vi "Basic Example.vi"() -> ()   [LabVIEW 2020]
uses:
  Laser Parameters.vi
panel:
  in  "REST port":string="35100"
  in  "Laser IP":string="10.0.40.83"
  in  "Ch2 Shutter":bool
  in  "Set Ch2 Wavl":bool
  in  "Ch2 Wavelength (nm)":dbl caption="Wavelength"
  in  "Ch1 Shutter":bool
  in  "Set Ch1 Wavl":bool
  in  "Ch1 Wavelength (nm)":dbl caption="Wavelength"
  in  "Ch3 Shutter":bool
  in  "stop":bool
  # "CRONUS-2P Laser Control Example\n\nA minimum working example of a CRONUS-2P\nlaser control application in LabVIEW.\n\nSet laser IP and REST port before running the\nprogram.\n\nTo change Ch1 or Ch2 wavelength, enter the value\nand press Set. The button will return to the false\nstate when wavelength setting is completed.\n\nToggle any of the shutter buttons to open or close\nthe output shutters.\n\nCopyright (c) 2018-2022 Light Conversion\n\nAll rights reserved.\n\nwww.lightcon.com"
  # "Channel 2"
  # "nm"
  # "Shutter"
  # "Channel 1"
  # "nm"
  # "Channel 3"
  # "1030 nm"
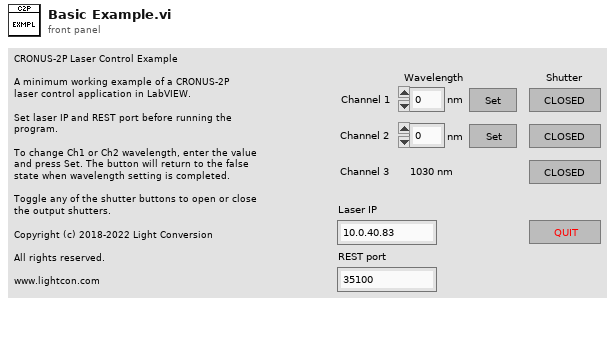
[diagram p1: front panel]
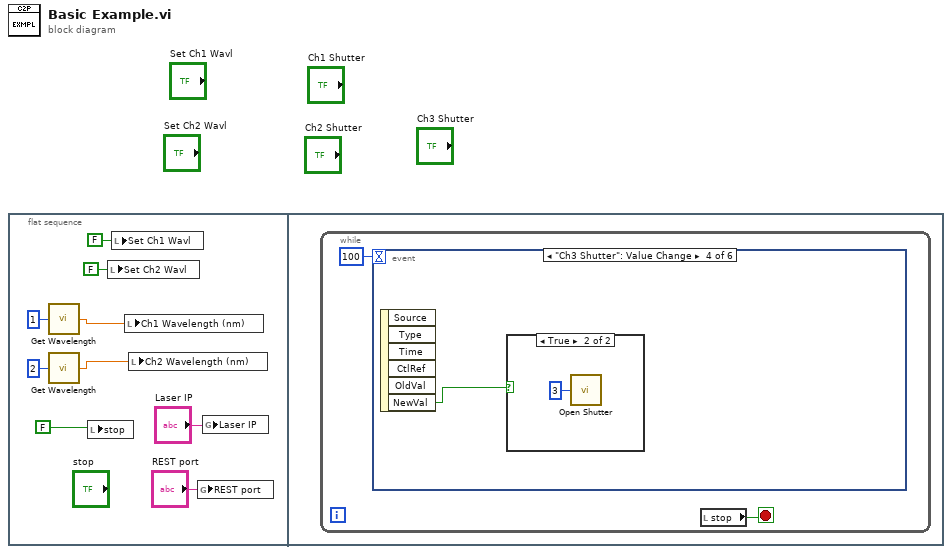
[diagram p0: block diagram]
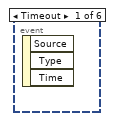
[diagram p2: hidden frame]
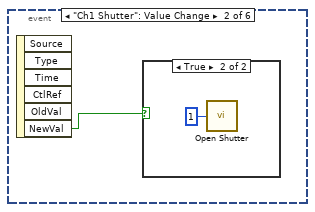
[diagram p3: hidden frame]
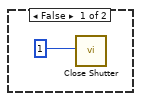
[diagram p4: hidden frame]
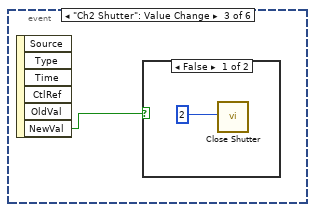
[diagram p5: hidden frame]
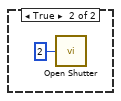
[diagram p6: hidden frame]
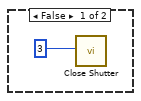
[diagram p7: hidden frame]
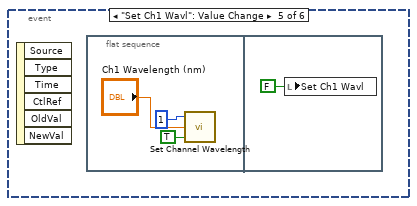
[diagram p8: hidden frame]
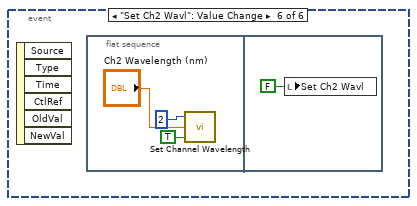
[diagram p9: hidden frame]
diagram:
  n1 = flat-sequence {
    frame #0 {
      n2 = call "Get Wavelength.vi"("Channel"=1) -> ("Wavelength (nm)"=w5:dbl)
      n3 = call "Get Wavelength.vi"("Channel"=2) -> ("Wavelength (nm)"=w6:dbl)
      n4 = local write "stop"(FALSE ("stop")) -> ()
      n5 = local write "Set Ch2 Wavl"(FALSE ("Set Ch2 Wavl")) -> ()
      n6 = local write "Set Ch1 Wavl"(FALSE ("Set Ch1 Wavl")) -> ()
      n7 = local write "Ch1 Wavelength (nm)"(w5) -> ()
      n8 = local write "Ch2 Wavelength (nm)"(w6) -> ()
      n9 = global write "Laser Parameters.vi" "REST port"("REST port") -> ()
      n10 = global write "Laser Parameters.vi" "Laser IP"("Laser IP") -> ()
    }
    frame #1 {
      n11 = while {
        stop <- w10 stop-if-true
        n12 = event shown="[3] \"Ch3 Shutter\": Value Change" {
          selector: _ -> [_ _ _ _ _ _]
          dyn-events: _ -> [_ _ _ _ _ _]
          timeout: 100 -> [_ _ _ _ _ _]
          event Timeout {
            n13 = event-data() -> ()  [unwired: 1 in, 3 out]
          }
          event "Ch1 Shutter": Value Change {
            n14 = event-data() -> ("NewVal"=w12:bool)  [unwired: 1 in, 5 out]
            n15 = case shown="True" w12 {
              frame False {
                n16 = call "Close Shutter.vi"("Channel"=1) -> ()  [unwired: 1 in]
              }
              frame True {
                n17 = call "Open Shutter.vi"("Channel"=1) -> ()  [unwired: 1 in]
              }
            }
          }
          event "Ch2 Shutter": Value Change {
            n18 = event-data() -> ("NewVal"=w15:bool)  [unwired: 1 in, 5 out]
            n19 = case shown="False" w15 {
              frame False {
                n20 = call "Close Shutter.vi"("Channel"=2) -> ()  [unwired: 1 in]
              }
              frame True {
                n21 = call "Open Shutter.vi"("Channel"=2) -> ()  [unwired: 1 in]
              }
            }
          }
          event "Ch3 Shutter": Value Change {
            n22 = event-data() -> ("NewVal"=w18:bool)  [unwired: 1 in, 5 out]
            n23 = case shown="True" w18 {
              frame False {
                n24 = call "Close Shutter.vi"("Channel"=3) -> ()  [unwired: 1 in]
              }
              frame True {
                n25 = call "Open Shutter.vi"("Channel"=3) -> ()  [unwired: 1 in]
              }
            }
          }
          event "Set Ch1 Wavl": Value Change {
            n26 = event-data() -> ()  [unwired: 1 in, 6 out]
            n27 = flat-sequence {
              frame #0 {
                n28 = call "Set Channel Wavelength.vi"("Wait until set"=TRUE, "Wavelength (nm)"="Ch1 Wavelength (nm)", "Channel"=1) -> ()  [unwired: 1 in]
              }
              frame #1 {
                n29 = local write "Set Ch1 Wavl"(FALSE ("Set Ch1 Wavl")) -> ()
              }
            }
          }
          event "Set Ch2 Wavl": Value Change {
            n30 = event-data() -> ()  [unwired: 1 in, 6 out]
            n31 = flat-sequence {
              frame #0 {
                n32 = call "Set Channel Wavelength.vi"("Wait until set"=TRUE, "Wavelength (nm)"="Ch2 Wavelength (nm)", "Channel"=2) -> ()  [unwired: 1 in]
              }
              frame #1 {
                n33 = local write "Set Ch2 Wavl"(FALSE ("Set Ch1 Wavl")) -> ()
              }
            }
          }
        }
        n34 = local read "stop"() -> (w10:bool)
      }
    }
  }
